vi "ingest.mcap.vi"(6 "Properties and Labels":T2, 7 "Locators":T1(array[cluster]), 8 "error in":errorcluster, 9 "Title and Description":cluster{"Title":string, "Description":string}, 10 "S3 Path":string, 11 "Nominal Client in":refnum<class "Nominal Client.lvclass">) -> (0 "error out":errorcluster, 1 "Response":T3, 2 "Video RID":string, 3 "Nominal Client out":refnum<class "Nominal Client.lvclass">, 4 "Response":string)   [LabVIEW 2020, in "Nominal Client.lvclass"]
doc: "<b> UNDER DEVELOPMENT! Do not use function </b>\n\nIngests data from mcap files in the S3 Nominal upload bucket. Currently only supports ingesting video channels."
uses:
  Nominal Client.lvclass
  4b965f09-dc68-4d5e-a5c1-32d476accfd4.vi
  03f47964-3351-4de7-ad21-2429850d9a88.vi
  328a2a72-b35c-448c-8cc8-7fb2a3abc54b.vi
  7ff8c0e1-378e-498f-a1ee-cc23b49038c3.vi
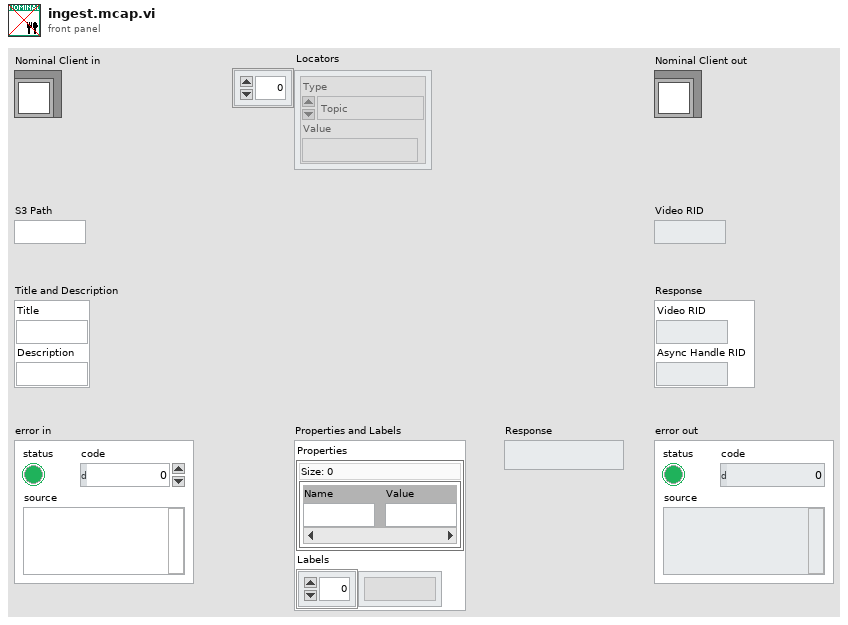
[diagram p1: front panel]
types:
  T1 = cluster{"Type":enum16{"Topic", "ID"}, "Value":string}[]
  T2 = cluster{"Properties":map{string, string}, "Labels":string[]}
  T3 = cluster{"Video RID":string, "Async Handle RID":string}
  T4 = cluster{"type":string, "s3":cluster{"path":string}}[]
  T5 = cluster{"type":string, "noManifest":cluster{"startingTimestamp":cluster{"secondsSinceEpoch":i32, "offsetNanoseconds":i32}}}
  T6 = cluster{"videoRid":string, "asyncHandle":cluster{"rid":string}}
  T7 = cluster{"type":string, "s3":cluster{"path":string}}
  T8 = cluster{"sources":cluster{"type":string, "s3":cluster{"path":string}}[], "properties":string, "labels":string[], "timestamps":cluster{"type":string, "noManifest":cluster{"startingTimestamp":cluster{"secondsSinceEpoch":i32, "offsetNanoseconds":i32}}}, "title":string, "description":string}
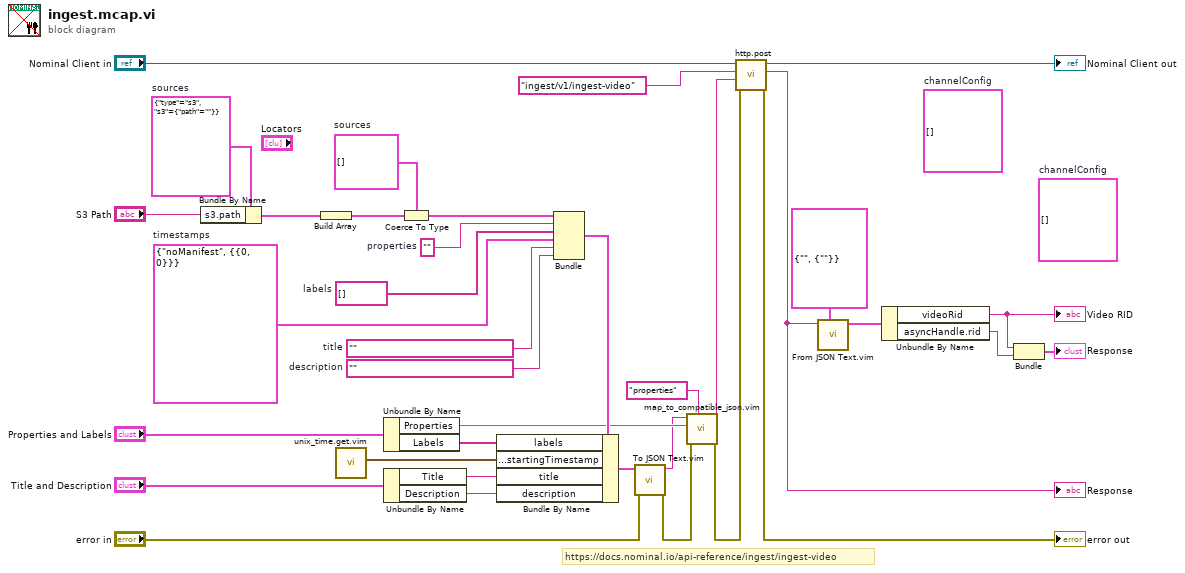
[diagram p0: block diagram]
diagram:
  (unwired) cluster{"type":string, "topic":string}[] []  # channelConfig
  (unwired) cluster{"type":string, "topic":string}[] []  # channelConfig
  w2 = T4 []  # sources
  w13 = ""  # properties
  w23 = ""  # description
  w24 = ""  # title
  w25 = T5 {"type"="noManifest", "noManifest"={"startingTimestamp"={"secondsSinceEpoch"=0, "offsetNanoseconds"=0}}}  # timestamps
  w26 = string[] []  # labels
  w7 = T7 {"type"="s3", "s3"={"path"=""}}  # sources
  # "https://docs.nominal.io/api-reference/ingest/ingest-video"
  n1 = Bundle By Name(cluster=w7, "s3.path"="S3 Path") -> (w5:T7)
  n2 = Build Array(w5) -> (w4:T4)
  n3 = call "unix_time.get.vim"() -> ("UNIX Timestamp"=w1:cluster{"Seconds":i64, "Nanoseconds":i64})  [unwired: 11 in]
  n4 = Unbundle By Name("Properties and Labels") -> ("Properties"=w14:map{string, string}, "Labels"=w18:string[])
  n5 = Unbundle By Name("Title and Description") -> ("Title"=w17:string, "Description"=w16:string)
  n6 = Coerce To Type(0:w4, 1:w2) -> (2:w3:T4)
  n7 = Bundle("sources"=w3, "properties"=w13, "labels"=w26, "timestamps"=w25, "title"=w24, "description"=w23) -> (w22:T8)  [unwired: 1 in]
  n8 = Bundle By Name(cluster=w22, "labels"=w18, "timestamps.noManifest.startingTimestamp"=w1, "title"=w17, "description"=w16) -> (w19:T8)
  n9 = call "To JSON Text.vim"("error in (no error)"="error in", "Anything"=w19) -> ("error out"=w9:errorcluster, "<JSON>"=w12:string)  [unwired: 8 in]
  n10 = call "map_to_compatible_json.vim"("JSON Path"="properties" ("Data Name"), "error in"=w9, "Map"=w14, "JSON in"=w12) -> ("error out"=w8:errorcluster, "JSON out"=w11:string)  [unwired: 6 in]
  n11 = call "http.post.vi"("error in"=w8, "Request body"=w11, "Path"="ingest/v1/ingest-video", "Nominal Client in"="Nominal Client in") -> ("error out"=→"error out":errorcluster, "Response"=w31:string, "Nominal Client out"=→"Nominal Client out":refnum<class "Nominal Client.lvclass">)  [unwired: 4 in, 1 out]
  "Response" <- w31
  n12 = call "From JSON Text.vim"("Data Type and Default Value"=T6 {"videoRid"="", "asyncHandle"={"rid"=""}} ("Information"), "JSON"=w31) -> ("Data out"=w30:T6)  [unwired: 8 in, 1 out]
  n13 = Unbundle By Name(w30) -> ("videoRid"=w29:string, "asyncHandle.rid"=w28:string)
  "Video RID" <- w29
  n14 = Bundle("videoRid"=w29, "rid"=w28) -> (→"Response":cluster{"videoRid":string, "rid":string})  [unwired: 1 in]
